vi "Get file group chan waveform.vi"(7 "Clip/desimate":T1={"Clip time"=FALSE, "Tiime 0"=0.0, "Time 1"=0.0, "Maximum data points"=1, "Decimation method"=enum."Min-Max"}, 8 "Error In":errorcluster, 9 "Channel":string, 10 "Group":string, 11 "File":path) -> (0 "Error Out":errorcluster, 3 "Waveform":waveform(sgl))   [LabVIEW 2015]
uses:
  Controls/Data reduction.ctl
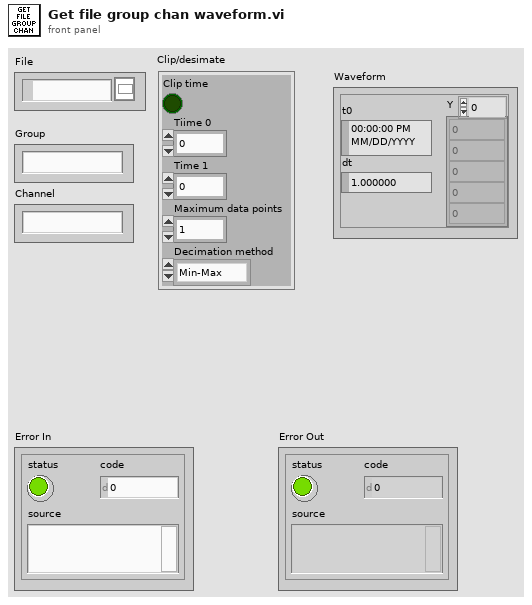
[diagram p1: front panel]
types:
  T1 = typedef "Data reduction.ctl" = cluster{"Clip time":bool, "Tiime 0":dbl, "Time 1":dbl, "Maximum data points":i32, "Decimation method":enum16{"coerce", "linear", "spline", "Min-Max", "Average"}}
  T2 = enum16{"open", "open or create", "create or replace", "create", "open (read-only)"}
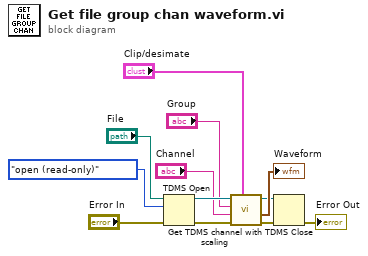
[diagram p0: block diagram]
diagram:
  n1 = TDMS Open(8:"Error In", 10:T2."open (read-only)" ("operation (0:open)"), 11:"File") -> (0:w5:errorcluster, 3:w8:refnum<k34>)  [unwired: 4 in]
  n2 = call "Get TDMS channel with scaling.vi"("Clip/desimate"="Clip/desimate", "error in"=w5, "Channel name"="Channel", "group name"="Group", "tdms file"=w8) -> ("error out"=w6:errorcluster, "output waveform"=→"Waveform":waveform(sgl), "tdms file out"=w7:refnum<k34>)  [unwired: 4 in]
  n3 = TDMS Close(8:w6, 11:w7) -> (0:→"Error Out":errorcluster)  [unwired: 1 out]
